vi "TestQueueTransport_ValueOK.vi"(8 "error in (no error)":errorcluster, 11 "TestCase in":refnum<class "TestTransport.lvclass">) -> (0 "error out":errorcluster, 3 "TestCase out":refnum<class "TestTransport.lvclass">)   [LabVIEW 2015, in "TestTransport.lvclass"]
uses:
  TestTransport.lvclass
  Framework/Mediator/Transport/QueueTransport/QueueTransport.lvclass
panel:
  out "element":T1
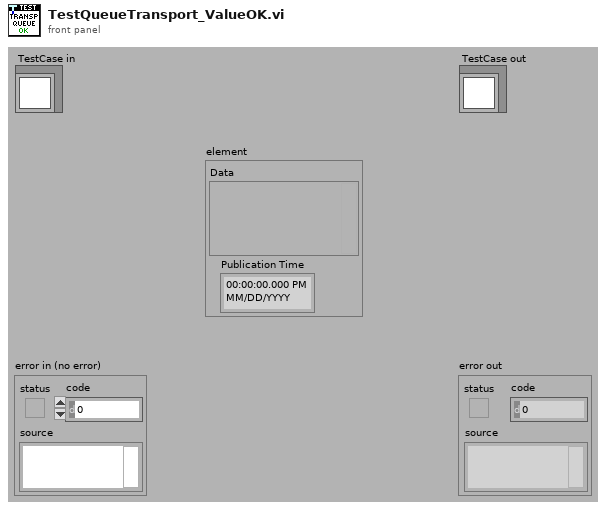
[diagram p1: front panel]
types:
  T1 = cluster{"Data":variant, "Publication Time":timestamp}
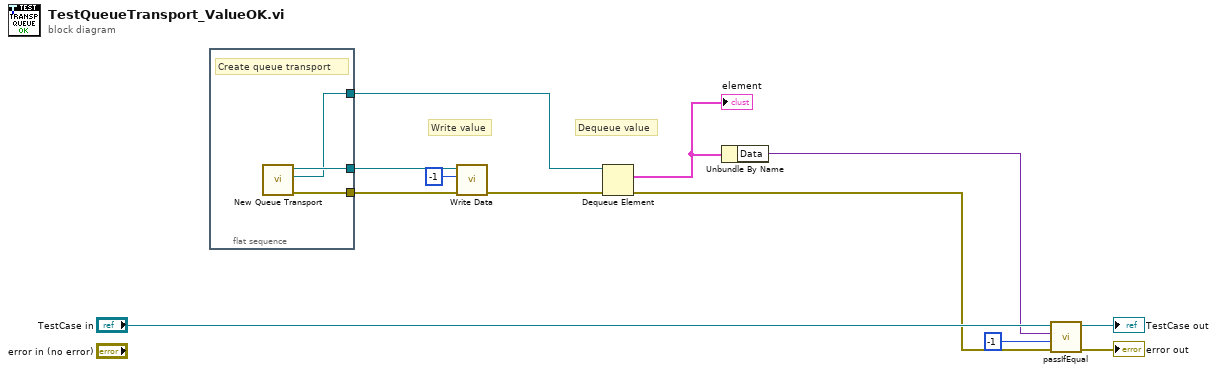
[diagram p0: block diagram]
diagram:
  # "Write value"
  # "Dequeue value"
  n1 = flat-sequence {
    tunnel: [w15] -> w7
    tunnel: [w14] -> w6
    tunnel: [w13] -> w3
    frame #0 {
      # "Create queue transport"
      n2 = call "New Queue Transport.vi"() -> ("error out"=w14:errorcluster, "Response Queue"=w13:refnum<queue>, "QueueTransport Out"=w15:refnum<class "QueueTransport.lvclass">)  [unwired: 9 in]
    }
  }
  n3 = call-dynamic "Write Data.vi"("error in (no error)"=w6, "Value"=-1, "QueueTransport In"=w7) -> ("error out"=w5:errorcluster)  [unwired: 7 in, 1 out]
  n4 = Dequeue Element(queue=w3, error in (no error)=w5) -> (element=w2:T1, error out=w4:errorcluster)  [unwired: 1 in, 2 out]
  "element" <- w2
  n5 = Unbundle By Name(w2) -> ("Data"=w1:variant)
  n6 = call-dynamic "passIfEqual.vi"("error in (no error)"=w4, "y"=-1, "x"=w1, "TestCase in"="TestCase in") -> ("error out"=→"error out":errorcluster, "TestCase out"=→"TestCase out":refnum<class "TestTransport.lvclass">)  [unwired: 6 in]
